vi "Ctrl.Bool.StyleFont.vi"(8 "error in (no error)":errorcluster, 10 "Font Info":T1, 11 "Bool Ref in":refnum<vi>) -> (0 "error out":errorcluster, 3 "Bool Ref out":refnum<vi>)   [LabVIEW 2017, in "JKI Simple Localization.lvlib"]
uses:
  API/JKI Simple Localization.lvlib
  Definitions/Private/Font Info.ctl
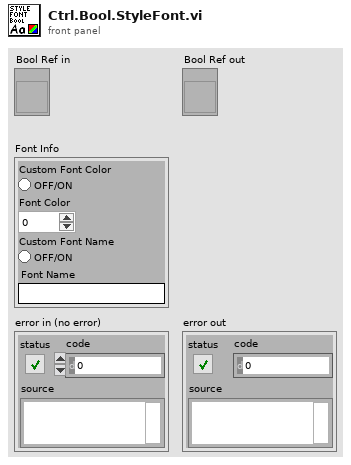
[diagram p1: front panel]
types:
  T1 = typedef "JKI Simple Localization.lvlib/Font Info.ctl" = cluster{"Custom Font Color":bool, "Font Color":u32, "Custom Font Name":bool, "Font Name":string}
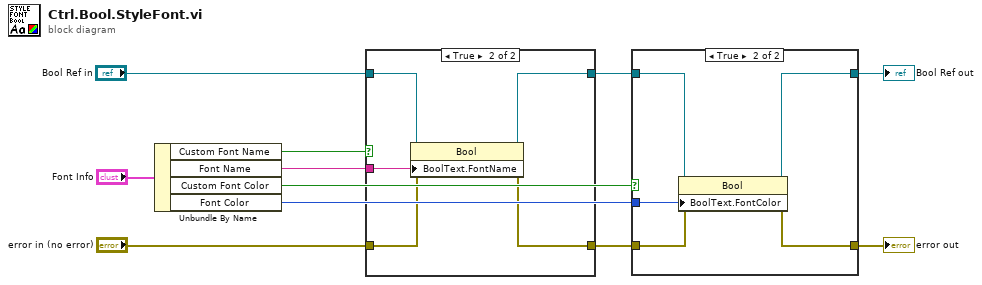
[diagram p0: block diagram]
diagram:
  n1 = Unbundle By Name("Font Info") -> ("Custom Font Name"=w10:bool, "Font Name"=w5:string, "Custom Font Color"=w8:bool, "Font Color"=w4:u32)
  n2 = case shown="True" w10 {
    tunnel: [w13 w17] -> w9
    tunnel: "error in (no error)" -> [w13 w18]
    tunnel: w5 -> [_ w14]
    tunnel: "Bool Ref in" -> [w12 w16]
    tunnel: [w12 w15] -> w2
    frame False {
    }
    frame True {
      n3 = property class="Bool"(reference=w16, error in=w18, "BoolText.FontName"=w14) -> (reference out=w15:refnum<vi>, error out=w17:errorcluster)
    }
  }
  n4 = case shown="True" w8 {
    tunnel: w9 -> [w20 w23]
    tunnel: [w20 w22] -> w6
    tunnel: w4 -> [_ w21]
    tunnel: w2 -> [w19 w25]
    tunnel: [w19 w24] -> w1
    frame False {
    }
    frame True {
      n5 = property class="Bool"(reference=w25, error in=w23, "BoolText.FontColor"=w21) -> (reference out=w24:refnum<vi>, error out=w22:errorcluster)
    }
  }
  "error out" <- w6
  "Bool Ref out" <- w1
